vi "ExCenterStripSpec.vi"() -> ()   [LabVIEW 2010]
panel:
  in  "Wavelength":dbl=546.0 format="%.2f"
  in  "Grating Speed":dbl=2000.0 min=1.0 step=1.0 format="%.2f"
  in  "Grating number":i16=1 min=1 max=100 step=1
  out "Strip":sgl[](graph)
  in  "Temperature":dbl=-10.0 format="%.2f"
  in  "Exposure":dbl=0.5 min=0.0 step=0.001 format="%.3f"
  in  "stop":bool
  out "error out":errorcluster
  in  "error in (no error)":errorcluster
  # "ExCenterStripSpec.vi\n(Normal Spectrograph via \nCOM/USB port)\nCamera and Spectrometer control.  This vi will open both the camera and spectrograph.  It will then move the grating to the Wavelength.  Data will then be collected and displayed until the STOP button is hit."
  # "NOTES:\nA properly configured camera .ini file may be required for camera operation.\n\nA properly configured spectrometer .ini file must be present in the LabVIEW folder for spectrograph operation.\n\nConsult the SITK documentation for more information on how to configure these files."
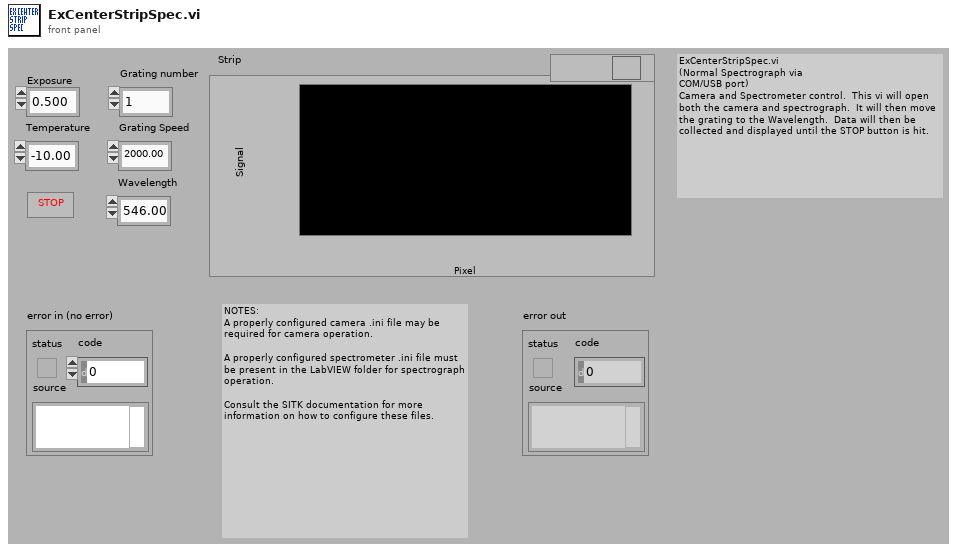
[diagram p1: front panel]
types:
  T1 = cluster{"acquire focus mode":u32, "Exposure":dbl, "Number of Images":u32, "Software accumulation":u32}
  T2 = cluster{"Camera Handle":u32, "Pulser Handle":u32, "File Handle":u32, "Display Handle":u32, "Image Handle":u32}
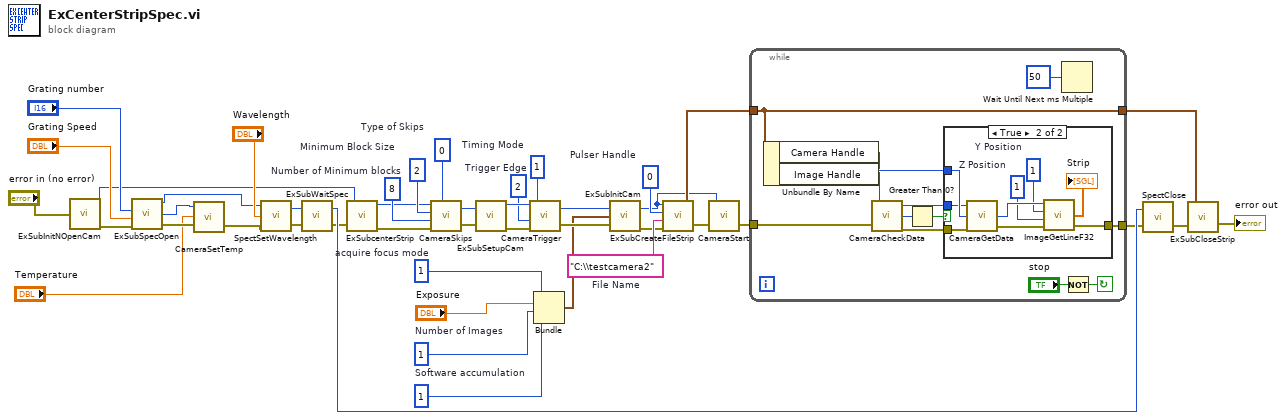
[diagram p0: block diagram]
diagram:
  w15 = u32 0  # Pulser Handle
  w20 = u32 1  # acquire focus mode
  w19 = u32 1  # Number of Images
  w18 = u32 1  # Software accumulation
  w17 = u32 1  # Timing Mode
  w21 = u32 2  # Trigger Edge
  w23 = u32 0  # Type of Skips
  w24 = u32 2  # Minimum Block Size
  w22 = u32 8  # Number of Minimum blocks
  w13 = "C:\\testcamera2"  # File Name
  n1 = call "ExSubInitNOpenCam.vi"("error in (no error)"="error in (no error)") -> ("Camera Handle"=w6:u32, "error out"=w33:errorcluster)
  n2 = call "ExSubSpecOpen.vi"("error in (no error)"=w33, "Grating speed"="Grating Speed", "Grating number"="Grating number") -> ("error out"=w5:errorcluster, "Camera Handle"=w2:u32, "Spectrometer Handle"=w1:u32)  [unwired: 1 in]
  n3 = call <userlib>:"CameraSetTemp.vi"("error in (no error)"=w5, "Temperature"="Temperature", "Camera Handle"=w2) -> ("error out"=w4:errorcluster)  [unwired: 1 out]
  n4 = call <userlib>:"SpectSetWavelength.vi"("error in"=w4, "Wavelength"="Wavelength", "Spectrometer Handle"=w1) -> ("error out"=w29:errorcluster, "Spectrumeter Handle"=w28:u32)
  n5 = call "ExSubWaitSpec.vi"("error in (no error)"=w29, "Spectrometer Handle"=w28) -> ("error out"=w12:errorcluster, "Spectrometer handle"=w26:u32)
  n6 = call "ExSubcenterStrip.vi"("error in (no error)"=w12, "Camera Handle"=w6) -> ("error out"=w10:errorcluster, "Camera Handle"=w11:u32)
  n7 = call <userlib>:"CameraSkips.vi"("Camera Handle"=w11, "Minimum Block Size"=w24, "Number of Minimum blocks"=w22, "error in"=w10, "Type of Skips"=w23) -> ("Camera Handle"=w36:u32, "error out"=w35:errorcluster)
  n8 = call "ExSubSetupCam.vi"("error in (no error)"=w35, "Camera Handle"=w36) -> ("error out"=w8:errorcluster, "Camera Handle"=w39:u32)
  n9 = call <userlib>:"CameraTrigger.vi"("error in"=w8, "Trigger Edge"=w21, "Timing Mode"=w17, "Camera Handle"=w39) -> ("error out"=w40:errorcluster, "Camera Handle"=w38:u32)
  n10 = Bundle("acquire focus mode"=w20, "Exposure"="Exposure", "Number of Images"=w19, "Software accumulation"=w18) -> (w16:T1)  [unwired: 1 in]
  n11 = call "ExSubInitCam.vi"("error in (no error)"=w40, "Camera Information"=w16, "Camera Handle"=w38) -> ("error out"=w9:errorcluster, "Camera Handle"=w14:u32)
  n12 = call "ExSubCreateFileStrip.vi"("error in (no error)"=w9, "File and Display Name"=w13, "Pulser Handle"=w15, "Camera Handle"=w14) -> ("error out"=w34:errorcluster, "Handles Out"=w42:T2)
  n13 = call <userlib>:"CameraStart.vi"("error in"=w34, "Camera Handle"=w14) -> ("error out"=w37:errorcluster)  [unwired: 1 out]
  n14 = while {
    tunnel: w42 -> [w53]
    tunnel: w37 -> [w52]
    tunnel: [w50] -> w25
    tunnel: [w53] -> w41
    stop <- w54 continue-if-true
    n15 = Unbundle By Name(w53) -> ("Camera Handle"=w45:u32, "Image Handle"=w49:u32)
    n16 = call <userlib>:"CameraCheckData.vi"("Camera Handle"=w45, "error in"=w52) -> ("Camera Handle"=w46:u32, "Number Of Frames Available"=w47:i32, "error out"=w51:errorcluster)
    n17 = Greater Than 0?(x=w47) -> (x > 0?=w48:bool)
    n18 = case shown="True" w48 {
      tunnel: w51 -> [w57 w65]
      tunnel: [w57 w63] -> w50
      tunnel: w49 -> [_ w61]
      tunnel: w46 -> [_ w60]
      frame False {
      }
      frame True {
        w58 = u32 1  # Z Position
        w59 = u32 1  # Y Position
        n19 = call <userlib>:"CameraGetData.vi"("error in"=w65, "Data Handle"=w61, "Camera Handle"=w60) -> ("error out"=w64:errorcluster, "Data Handle"=w62:u32)  [unwired: 1 out]
        n20 = call <userlib>:"ImageGetLineF32.vi"("error in"=w64, "Z Position"=w58, "Y Position"=w59, "Data Handle"=w62) -> ("error out"=w63:errorcluster, "Array F32"=→"Strip":sgl[])  [unwired: 1 out]
      }
    }
    n21 = Wait Until Next ms Multiple(millisecond multiple=u32 50) -> ()  [unwired: 1 out]
    n22 = Not(x="stop") -> (.not. x?=w54:bool)
  }
  n23 = call <userlib>:"SpectClose.vi"("error in"=w25, "Spectrometer Handle"=w26) -> ("error out"=w27:errorcluster)
  n24 = call "ExSubCloseStrip.vi"("error in (no error)"=w27, "Handles In"=w41) -> ("error out"=→"error out":errorcluster)
